vi "RegisterCallback.vi"(8 "error in (no error)":errorcluster, 10 "Menu Item":refnum<k24>, 11 "MGI_TrayIcon in":refnum<class "MGI_TrayIcon.lvclass">) -> (0 "error out":errorcluster, 3 "MGI_TrayIcon out":refnum<class "MGI_TrayIcon.lvclass">)   [LabVIEW 2016, in "MGI_TrayIcon.lvclass"]
doc: "Registers for the menu item clicked event.\n\nAuthored by Derek E. Trepanier\nsupport@mooregoodideas.com\nwww.mooregoodideas.com\n\nCopyright (c) 2012, Moore Good Ideas, Inc.\n\nAll rights reserved.\n\nRedistribution and use in source and binary forms, with or without modification, are permitted provided that the following conditions are met:\n\n * Redistributions of source code must retain the above copyright notice, this list of conditions and the following disclaimer.\n * Redistributions in binary form must reproduce the above copyright notice, this list of conditions and the following disclaimer in the documentation and/or other materials provided with the distribution.\n * Neither the name of Moore Good Ideas, Inc. nor the names of its contributors may be used to endorse or promote products derived from this software without specific prior written permission.\n\nTHIS SOFTWARE IS PROVIDED BY THE COPYRIGHT HOLDERS AND CONTRIBUTORS \"AS IS\" AND ANY EXPRESS OR IMPLIED WARRANTIES, INCLUDING, BUT NOT LIMITED TO, THE IMPLIED WARRANTIES OF MERCHANTABILITY AND FITNESS FOR A PARTICULAR PURPOSE ARE DISCLAIMED. IN NO EVENT SHALL THE COPYRIGHT OWNER OR CONTRIBUTORS BE LIABLE FOR ANY DIRECT, INDIRECT, INCIDENTAL, SPECIAL, EXEMPLARY, OR CONSEQUENTIAL DAMAGES (INCLUDING, BUT NOT LIMITED TO, PROCUREMENT OF SUBSTITUTE GOODS OR SERVICES; LOSS OF USE, DATA, OR PROFITS; OR BUSINESS INTERRUPTION) HOWEVER CAUSED AND ON ANY THEORY OF LIABILITY, WHETHER IN CONTRACT, STRICT LIABILITY, OR TORT (INCLUDING NEGLIGENCE OR OTHERWISE) ARISING IN ANY WAY OUT OF THE USE OF THIS SOFTWARE, EVEN IF ADVISED OF THE POSSIBILITY OF SUCH DAMAGE."
uses:
  <userlib>/_MGI/Menu Building/MenuTypes/TrayIcon/MGI_TrayIcon.lvclass
  System.Windows.Forms
  <userlib>/_MGI/Menu Building/MenuTypes/TrayIcon/MGI_TrayIcon.lvclass/MGI_TrayIcon.ctl
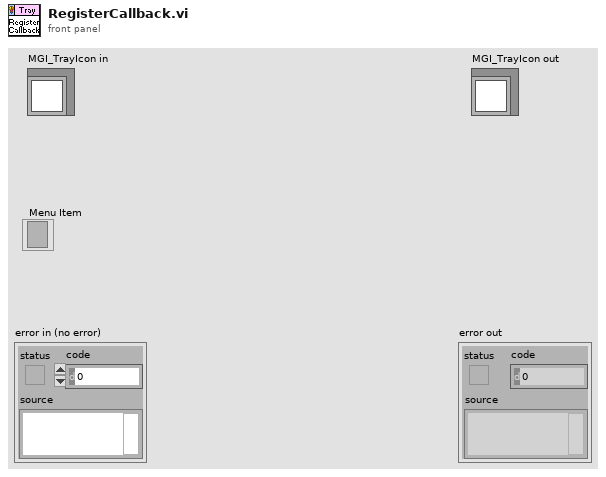
[diagram p1: front panel]
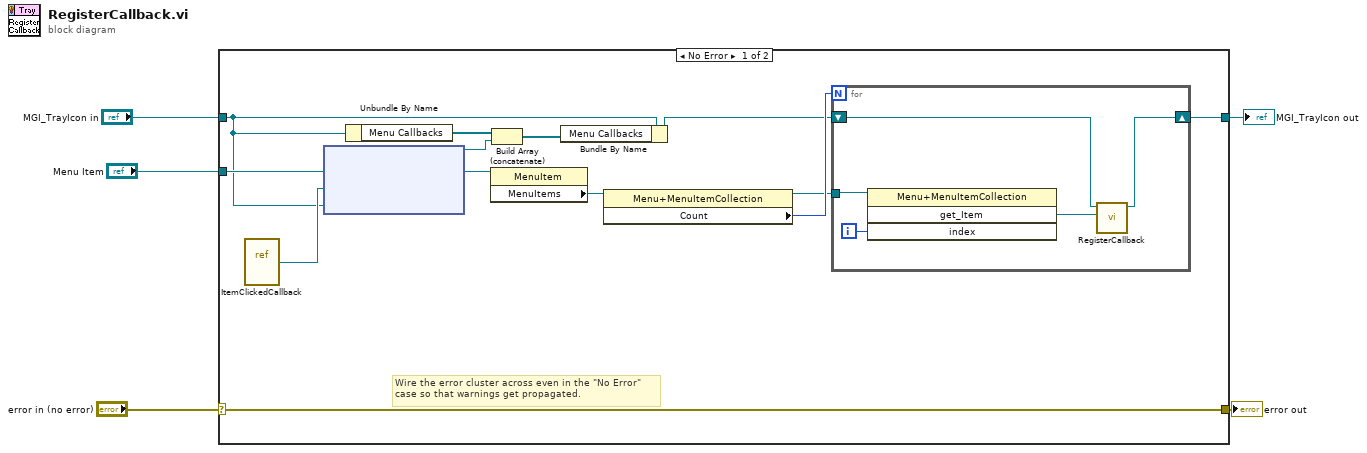
[diagram p0: block diagram]
diagram:
  n1 = case shown="No Error" "error in (no error)" {
    selector: "error in (no error)" -> [w17 w24]
    tunnel: [w17 w24] -> w4
    tunnel: "Menu Item" -> [w16 _]
    tunnel: "MGI_TrayIcon in" -> [w10 w23]
    tunnel: [w13 w23] -> w1
    frame No Error {
      # "Wire the error cluster across even in the \"No Error\"\ncase so that warnings get propagated."
      n2 = vi-ref <userlib>:"ItemClickedCallback.vi"() -> ("vi reference"=w15:refnum<vi>)
      n3 = node(w16, w15, w10) -> (w8:refnum<k27>)  [unwired: 2 in, 1 out]
      n4 = Unbundle By Name(w10) -> ("Menu Callbacks"=w9:refnum<k27>[])
      n5 = property class="MenuItem"(reference=w16) -> ("MenuItems"=w14:refnum<k24>)  [unwired: 1 in, 2 out]
      n6 = Build Array (concatenate)(w9, w8) -> (w6:refnum<k27>[])
      n7 = Bundle By Name(cluster=w10, "Menu Callbacks"=w6) -> (w7:refnum<class "MGI_TrayIcon.lvclass">)
      n8 = property class="Menu+MenuItemCollection"(reference=w14) -> (reference out=w11:refnum<k24>, "Count"=w12:i32)  [unwired: 1 in, 1 out]
      n9 = for {
        N: w12 -> [_]
        tunnel: w11 -> [w22]
        shift-right: [w19] -> w13
        shift-left: w7 -> [w20]
        i -> [w21]
        n10 = invoke class="Menu+MenuItemCollection" method="get_Item"(reference=w22, "index"=w21) -> ("get_Item"=w18:refnum<k24>)  [unwired: 2 in, 3 out]
        n11 = call <userlib>:"RegisterCallback.vi"("Menu Item"=w18, "MGI_TrayIcon in"=w20) -> ("MGI_TrayIcon out"=w19:refnum<class "MGI_TrayIcon.lvclass">)  [unwired: 8 in, 1 out]
      }
    }
    frame Error {
    }
  }
  "error out" <- w4
  "MGI_TrayIcon out" <- w1
